vi "t1.vi"(11 "C":dbl) -> (3 "Numeric":dbl)   [LabVIEW 2015]
doc: "yo"
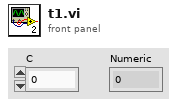
[diagram p1: front panel]
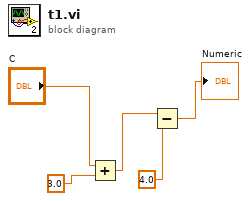
[diagram p0: block diagram]
diagram:
  n1 = Add(x="C", y=3.0 ("x+y")) -> (x+y=w3:dbl)
  n2 = Subtract(x=w3, y=4.0 ("x-y")) -> (x-y=→"Numeric":dbl)
